vi "Initialize Rx Channel.vi"(8 "error in":errorcluster, 9 "channel speed":u32(ring) items=["API429_LO_SPEED", "API429_HI_SPEED"], 10 "channel number":u8, 11 "board handle":u8) -> (0 "error out":errorcluster, 2 "channel number out":u8, 3 "board handle out":u8)   [LabVIEW 2020, in "AIM ARINC 429 Hardware API.lvlib"]
uses:
  AIM ARINC 429 Hardware API.lvlib
  Channel Action.ctl
  <instrlib>/AIM GmbH/_ARINC-429/AIM429LV.lvlib
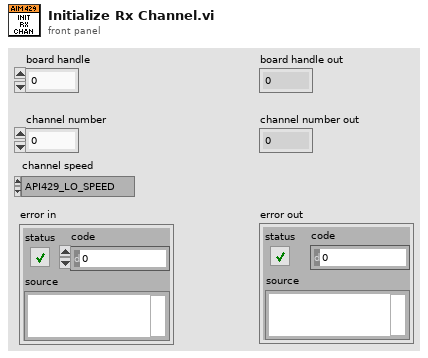
[diagram p1: front panel]
types:
  T1 = typedef "AIM ARINC 429 Hardware API.lvlib/Channel Action.ctl" = enum16{"Get Info", "Initialize", "Start", "Clear"}
  T2 = typedef "AIM ARINC 429 Hardware API.lvlib/Channel Status.ctl" = enum16{"Uninitialized", "Idle", "Active"}
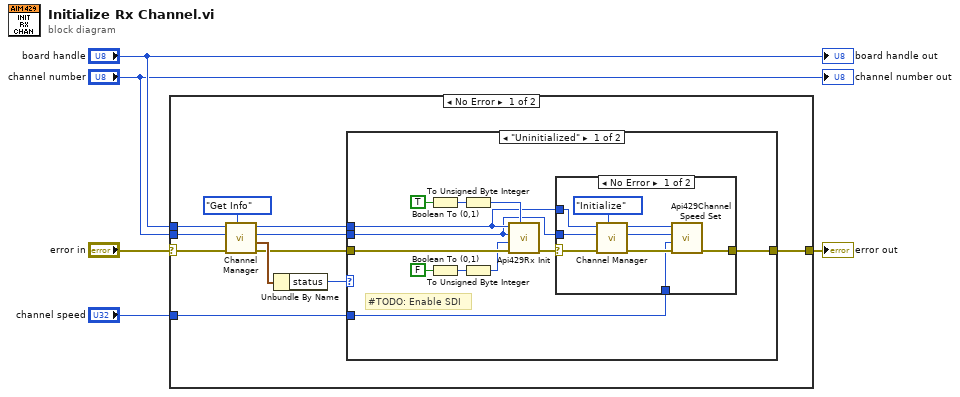
[diagram p0: block diagram]
diagram:
  n1 = case shown="No Error" "error in" {
    selector: "error in" -> [w8 w40]
    tunnel: "board handle" -> [w16 _]
    tunnel: "channel number" -> [w15 _]
    tunnel: [w7 w40] -> w2
    tunnel: "channel speed" -> [w6 _]
    frame No Error {
      n2 = call "Channel Manager.vi"("action"=Channel_Action."Get Info", "error in"=w8, "channel number"=w15, "board handle"=w16) -> ("error out"=w11:errorcluster, "channel info"=w13:cluster{"count":u32, "status":T2}, "channel number out"=w9:u8, "board handle out"=w10:u8)  [unwired: 4 in]
      n3 = Unbundle By Name(w13) -> ("status"=w12:T2)
      n4 = case shown="\"Uninitialized\"" w12 {
        tunnel: w11 -> [w28 w39]
        tunnel: w10 -> [w19 _]
        tunnel: w9 -> [w18 _]
        tunnel: [w20 w39] -> w7
        tunnel: w6 -> [w17 _]
        frame "Uninitialized" {
          # "#TODO: Enable SDI"
          n5 = Boolean To (0,1)(Boolean=TRUE) -> (0, 1=w24:i16)
          n6 = Boolean To (0,1)(Boolean=FALSE) -> (0, 1=w26:i16)
          n7 = To Unsigned Byte Integer(number=w24) -> (unsigned 8bit integer=w22:u8)
          n8 = To Unsigned Byte Integer(number=w26) -> (unsigned 8bit integer=w25:u8)
          n9 = call <instrlib>:"Api429Rx Init.vi"("parity_check_enabled"=w22, "error in (no error)"=w28, "sdi_enabled"=w25, "b_Chn"=w18, "board_handle"=w19) -> ("error out"=w21:errorcluster)  [unwired: 6 in]
          n10 = case shown="No Error" w21 {
            selector: w21 -> [w36 w38]
            tunnel: [w32 w38] -> w20
            tunnel: w19 -> [w35 _]
            tunnel: w18 -> [w34 _]
            tunnel: w17 -> [w29 _]
            frame No Error {
              n11 = call "Channel Manager.vi"("action"=Channel_Action."Initialize", "error in"=w36, "channel number"=w34, "board handle"=w35) -> ("error out"=w33:errorcluster, "channel number out"=w30:u8, "board handle out"=w31:u8)  [unwired: 4 in, 1 out]
              n12 = call <instrlib>:"Api429Channel Speed Set.vi"("error in (no error)"=w33, "speed"=w29, "b_Chn"=w30, "board_handle"=w31) -> ("error out"=w32:errorcluster)  [unwired: 7 in]
            }
            frame Error {
            }
          }
        }
        frame Default {
          # "channel is already initialized; don't call init again"
        }
      }
    }
    frame Error {
    }
  }
  "error out" <- w2
  "board handle out" <- "board handle"
  "channel number out" <- "channel number"
